vi "TCP-Send Command Receive String.vi"(0 "PXI Address":string, 5 "Port":i32, 7 "Command":string, 9 "timeout (ms)":i32=5000, 11 "error in (no error)":errorcluster, 12 "byte order":T1(ring)=enum."native, host order") -> (4 "data":string, 15 "error out":errorcluster)   [LabVIEW 2020]
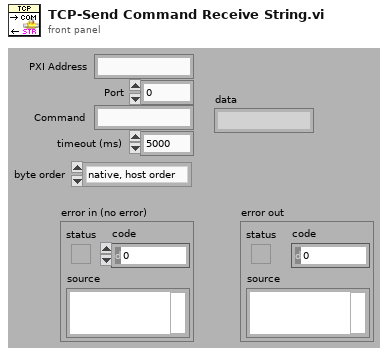
[diagram p1: front panel]
types:
  T1 = enum16{"big-endian, network order", "native, host order", "little-endian"}
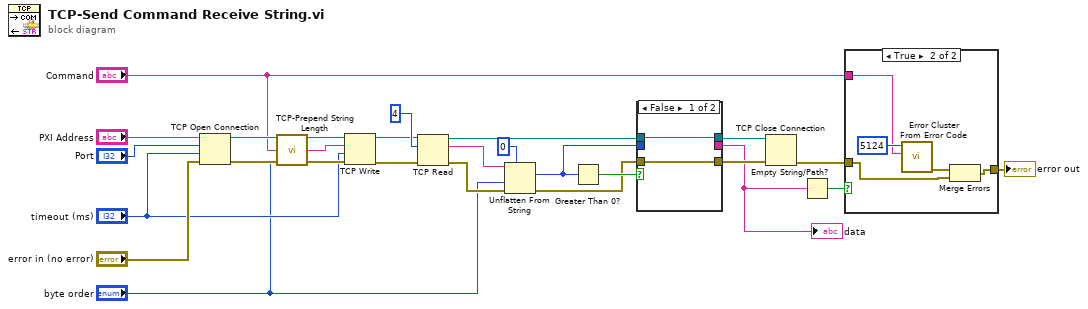
[diagram p0: block diagram]
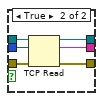
[diagram p2: hidden frame]
diagram:
  n1 = TCP Open Connection(address="PXI Address", remote port or service name="Port", timeout ms (60000)="timeout (ms)", error in (no error)="error in (no error)") -> (connection ID=w21:refnum<k5>, error out=w22:errorcluster)  [unwired: 1 in]
  n2 = call "TCP-Prepend String Length.vi"("byte order"="byte order", "Command"="Command") -> ("String"=w8:string)  [unwired: 3 in]
  n3 = TCP Write(connection ID=w21, data in=w8, error in (no error)=w22, 9:"timeout (ms)") -> (connection ID out=w16:refnum<k5>, error out=w15:errorcluster)  [unwired: 1 out]
  n4 = TCP Read(connection ID=w16, bytes to read=4, error in (no error)=w15) -> (connection ID out=w14:refnum<k5>, data out=w5:string, error out=w3:errorcluster)  [unwired: 2 in]
  n5 = Unflatten From String(type=0, binary string=w5, byte order (0:big-endian, network order)="byte order", error in (no error)=w3) -> (value=w4:i32, error out=w2:errorcluster)  [unwired: 1 in, 1 out]
  n6 = Greater Than 0?(x=w4) -> (x > 0?=w12:bool)
  n7 = case shown="False" w12 {
    tunnel: [_ w33] -> w9
    tunnel: [w27 w32] -> w11
    tunnel: w14 -> [w26 w31]
    tunnel: w2 -> [w27 w30]
    tunnel: w4 -> [_ w29]
    tunnel: [w26 w28] -> w13
    frame False {
    }
    frame True {
      n8 = TCP Read(connection ID=w31, bytes to read=w29, error in (no error)=w30) -> (connection ID out=w28:refnum<k5>, data out=w33:string, error out=w32:errorcluster)  [unwired: 2 in]
    }
  }
  "data" <- w9
  n9 = TCP Close Connection(connection ID=w13, error in (no error)=w11) -> (error out=w18:errorcluster)  [unwired: 1 in, 1 out]
  n10 = Empty String/Path?(string/path=w9) -> (empty?=w10:bool)
  n11 = case shown="True" w10 {
    tunnel: [w34 w36] -> w19
    tunnel: w18 -> [w34 w35]
    tunnel: "Command" -> [_ w37]
    frame False {
    }
    frame True {
      n12 = call <vilib>:"Error Cluster From Error Code.vi"("error message (\"\")"=w37, "error code (0)"=5124) -> ("error out"=w39:errorcluster)  [unwired: 7 in]
      n13 = Merge Errors(w39, w35) -> (w36:errorcluster)
    }
  }
  "error out" <- w19
